vi "Write2Markdown.vi"(0 "String":string) -> ()   [LabVIEW 2019]
panel:
  out "date/time string":string
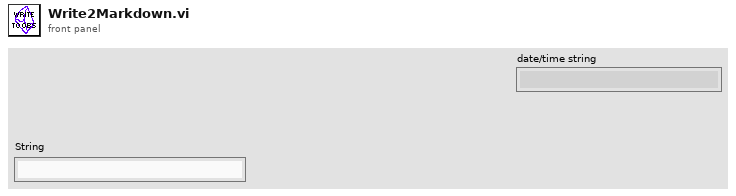
[diagram p1: front panel]
types:
  T1 = enum16{"open", "replace", "create", "open or create", "replace or create", "replace or create with confirmation"}
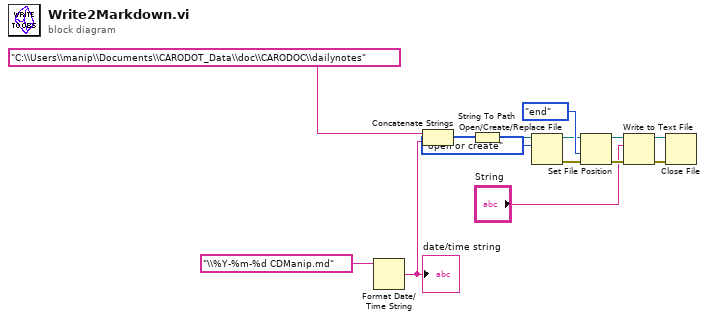
[diagram p0: block diagram]
diagram:
  n1 = Format Date/Time String(time format string (%c)="\\%Y-%m-%d CDManip.md") -> (date/time string=w5:string)  [unwired: 2 in]
  "date/time string" <- w5
  n2 = Concatenate Strings("C:\\Users\\manip\\Documents\\CARODOT_Data\\doc\\CARODOC\\dailynotes", w5) -> (w4:string)
  n3 = String To Path(string=w4) -> (path=w3:path)
  n4 = Open/Create/Replace File(file path (use dialog)=w3, operation (0:open)=T1."open or create") -> (refnum out=w13:refnum<file>, error out=w8:errorcluster)  [unwired: 4 in, 1 out]
  n5 = Set File Position(refnum=w13, from (0:start)=enum16{"start", "end", "current"}."end", error in=w8) -> (refnum out=w12:refnum<file>, error out=w9:errorcluster)  [unwired: 1 in]
  n6 = Write to Text File(file (use dialog)=w12, text="String", error in=w9) -> (refnum out=w11:refnum<file>, error out=w10:errorcluster)  [unwired: 1 in, 1 out]
  n7 = Close File(refnum=w11, error in=w10) -> ()  [unwired: 2 out]
